vi "Read Param.vi"(8 "error in (no error)":errorcluster, 11 "Param in":T1) -> (0 "error out":errorcluster, 2 "PAR":dbl[][](array[numeric]), 3 "Param out":T1)   [LabVIEW 2019, in "Inputs.lvlib"]
uses:
  Inputs.lvlib
  Ctl/Param.ctl
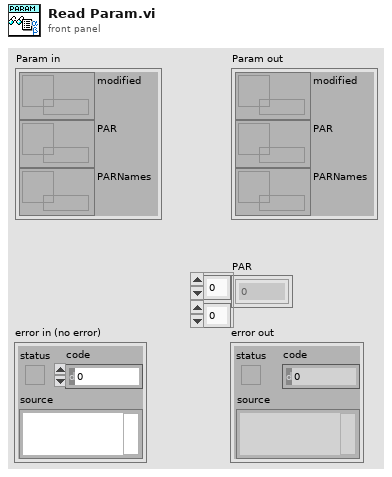
[diagram p1: front panel]
types:
  T1 = typedef "Inputs.lvlib/Param.ctl" = cluster{"modified":refnum<data-value>, "PAR":refnum<data-value>, "PARNames":refnum<data-value>}
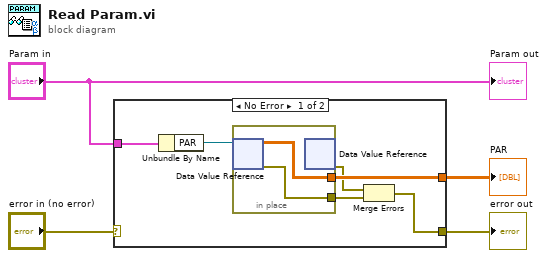
[diagram p0: block diagram]
diagram:
  n1 = case shown="No Error" "error in (no error)" {
    selector: "error in (no error)" -> [_ w13]
    tunnel: [w6 w13] -> w1
    tunnel: "Param in" -> [w5 _]
    tunnel: [w9 _] -> w2
    frame No Error {
      n2 = Unbundle By Name(w5) -> ("PAR"=w10:refnum<data-value>)
      n3 = in-place {
        in-place-border: [w12] -> w8
        in-place-border: [w11] -> w9
        n4 = in-place-dvr #1(w10) -> (w11:dbl[][], w12:errorcluster)
        n5 = in-place-dvr #1() -> (w7:errorcluster)  [unwired: 1 in, 1 out]
      }
      n6 = Merge Errors(w7, w8) -> (w6:errorcluster)
    }
    frame Error {
    }
  }
  "error out" <- w1
  "PAR" <- w2
  "Param out" <- "Param in"
